vi "Ex_03 Monitor.vi"(0 "VISA resource name":refnum<visa-resource-name>="COM1", 1 "baud rate":u32=9600, 2 "data bits":u16=8 min=5 max=8 step=1, 3 "parity":u16(ring) items=["None", "Odd", "Even", "Mark", "Space"], 4 "stop bits":u16(ring)=10 items=["1.0"=10, "1.5"=15, "2.0"=20], 6 "read":bool=TRUE, 7 "flow control":u16(ring) items=["None"=0, "XON/XOFF"=1, "RTS/CTS"=2, "DTR/DSR"=4]) -> (9 "read string":string, 10 "bytes read":u32)   [LabVIEW 2010]
doc: "The Basic Serial Read and Write example performs a Serial Port Read, a Serial Port Write, or a combination of these actions. The user selects the actions (read or write) on the front panel. If both are selected, the VI will write the data first, read data, and then close the VISA session that is opened to the port. This VI will wait until the specified number of bytes is received at the port or until a termination character is read.\n\nINSTRUCTIONS:\n1) Select the serial resource and configuration parameters (baud rate, data bits, parity, stop bits, flow control).\n2) Select the operations to be performed. \n3) Connect the serial port to your device. If no device is available, perform a loopback test by doing one of the following. Short pins 2 and 3 on a RS-232 cable or short pin 4 to pin 8 and pin 5 to pin 9 on a RS-485/422 cable. \n4) Run the VI to see the data read. (The \"read string\" will match the \"string to write\" if a loopback test was performed.)\n\nNote: The parameters set for the serial port must match the parameters of the connected instrument or device. In this example, the bytes to read parameter specifies the number of bytes that the serial port reads. If there were more bytes at the port than the number specified in bytes to read, those bytes would not be read. Also, if you specify to read more bytes than the number of bytes actually read, you might receive a timeout error message.\n\nOn the block diagram, the Configure Serial Port VI sets the configuration parameters. The front panel displays the controls used to configure the basic parameters, such as baud rate, data bits, and parity. Constants configure the other parameters the user probably does not need set. After the VISA Configure Serial Port VI opens the VISA session and configures the port, the VI passes the VISA resource name to other VIs that perform operations on that VISA resource. The VISA Write function sends a command to the serial device and the VISA Read function returns data based on the command. The VISA Close function then closes the reference to the serial device. It is important to close the reference; otherwise communication through with that port through protocols other than VISA might not be possible."
uses:
  <vilib>/Instr/_visa.llb/VISA Configure Serial Port (Instr).vi
panel:
  in  "stop":bool
  out "Meter":dbl(knob) scale=0.0..1024.0
  out "read string 2":string
  in  "On":bool
  in  "Off":bool
  in  "delay before read (ms)":u32=500
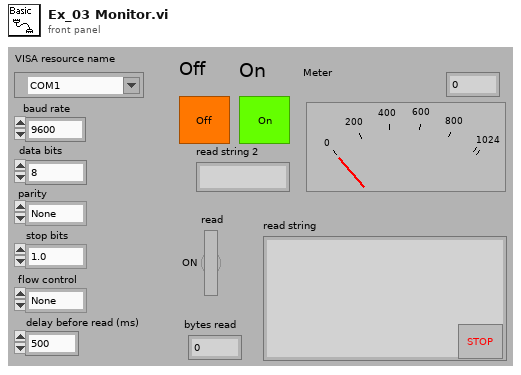
[diagram p1: front panel]
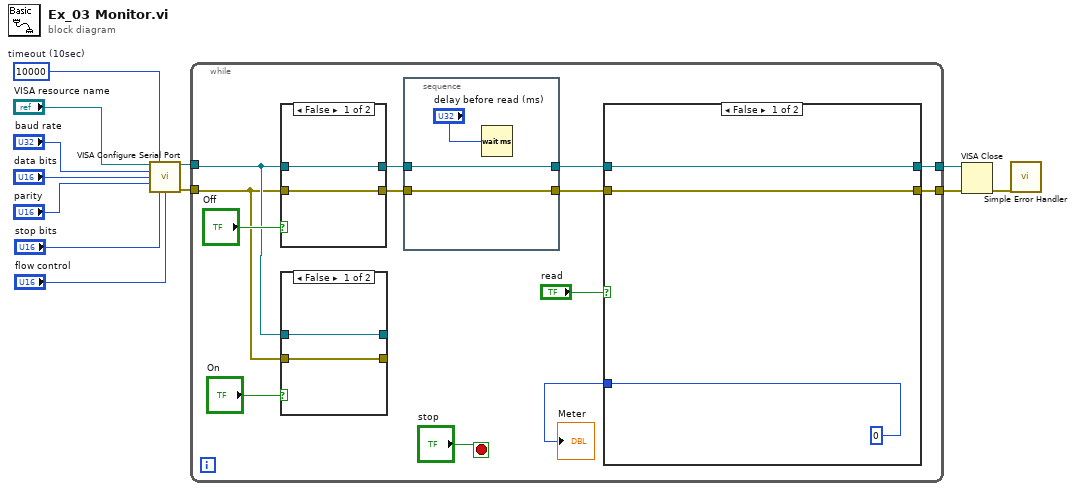
[diagram p0: block diagram]
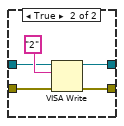
[diagram p2: hidden frame]
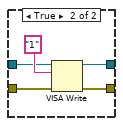
[diagram p3: hidden frame]
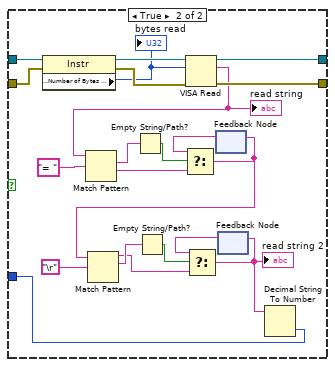
[diagram p4: hidden frame]
diagram:
  w8 = u32 10000  # timeout (10sec)
  n1 = call-poly "VISA Configure Serial Port"("VISA resource name"="VISA resource name", "timeout (10sec)"=w8, "baud rate (9600)"="baud rate", "data bits (8)"="data bits", "parity (0:none)"="parity", "stop bits (10: 1 bit)"="stop bits", "flow control (0:none)"="flow control") -> ("VISA resource name out"=w3:refnum<visa-resource-name>, "error out"=w4:errorcluster)  [unwired: 2 in, 5 out]
  n2 = while {
    tunnel: w3 -> [w17]
    tunnel: w4 -> [w16]
    tunnel: [w15] -> w2
    tunnel: [w14] -> w1
    stop <- "stop" stop-if-true
    n3 = case shown="False" "Off" {
      tunnel: [w37 w42] -> w19
      tunnel: w17 -> [w36 w40]
      tunnel: w16 -> [w37 w39]
      tunnel: [w36 w38] -> w21
      frame False {
      }
      frame True {
        n4 = VISA Write(VISA resource name=w40, write buffer="1" ("string to write"), error in (no error)=w39) -> (VISA resource name out=w38:refnum<visa-resource-name>, error out=w42:errorcluster)  [unwired: 1 out]
      }
    }
    n5 = case shown="False" "On" {
      tunnel: [w27 w32] -> _
      tunnel: w17 -> [w26 w30]
      tunnel: w16 -> [w27 w29]
      tunnel: [w26 w28] -> _
      frame False {
      }
      frame True {
        n6 = VISA Write(VISA resource name=w30, write buffer="2" ("string to write"), error in (no error)=w29) -> (VISA resource name out=w28:refnum<visa-resource-name>, error out=w32:errorcluster)  [unwired: 1 out]
      }
    }
    n7 = stacked-sequence {
      tunnel: w19 -> [w35]
      tunnel: [w35] -> w20
      tunnel: w21 -> [w34]
      tunnel: [w34] -> w22
      frame #0 {
        n8 = Wait (ms)(milliseconds to wait="delay before read (ms)") -> ()  [unwired: 1 out]
      }
    }
    n9 = case shown="False" "read" {
      tunnel: w20 -> [w45 w62]
      tunnel: [w45 w66] -> w14
      tunnel: [w44 w65] -> w15
      tunnel: w22 -> [w44 w64]
      tunnel: [0 w46] -> w13
      frame False {
      }
      frame True {
        n10 = property class="Instr"(reference=w64, error in=w62) -> (reference out=w63:refnum<visa-resource-name>, error out=w61:errorcluster, "Serial Settings:Number of Bytes at Serial Port"=w60:u32)
        "bytes read" <- w60
        n11 = VISA Read(VISA resource name=w63, byte count=w60, error in (no error)=w61) -> (VISA resource name out=w65:refnum<visa-resource-name>, read buffer=w54:string, error out=w66:errorcluster)  [unwired: 1 out]
        "read string" <- w54
        n12 = Match Pattern(string=w54, regular expression="= ") -> (match substring=w57:string, after substring=w56:string)  [unwired: 3 out]
        n13 = Empty String/Path?(string/path=w57) -> (empty?=w59:bool)
        n14 = feedback #1() -> (w58:string)  [unwired: 1 out]
        n15 = Select(t=w58, s=w59, f=w56) -> (s? t:f=w51:string)
        n16 = Match Pattern(string=w51, regular expression="\r") -> (before substring=w48:string, match substring=w49:string)  [unwired: 3 out]
        n17 = Empty String/Path?(string/path=w49) -> (empty?=w53:bool)
        n18 = feedback-in #1(w51) -> ()
        n19 = feedback #2() -> (w52:string)  [unwired: 1 out]
        n20 = Select(t=w52, s=w53, f=w48) -> (s? t:f=w47:string)
        "read string 2" <- w47
        n21 = feedback-in #2(w47) -> ()
        n22 = Decimal String To Number(string=w47) -> (number=w46:i32)  [unwired: 2 in, 1 out]
      }
    }
    "Meter" <- w13
  }
  n23 = VISA Close(VISA resource name=w2, error in (no error)=w1) -> (error out=w10:errorcluster)
  n24 = call <vilib>:"Simple Error Handler.vi"("error in (no error)"=w10) -> ()  [unwired: 1 in, 8 out]
